vi "Test Normalise.vi"(11 "Test Case In":refnum<class "Vector 2D Tests.lvclass">) -> (0 "error out":errorcluster, 3 "Test Case Out":refnum<class "Vector 2D Tests.lvclass">)   [LabVIEW 2021, in "Vector 2D Tests.lvclass"]
uses:
  Vector 2D Tests.lvclass
  4993e8ee-a06a-463a-9684-69129f64d5ce.vi
  Re-use Libraries/Vector 2D/Vector 2D.lvclass
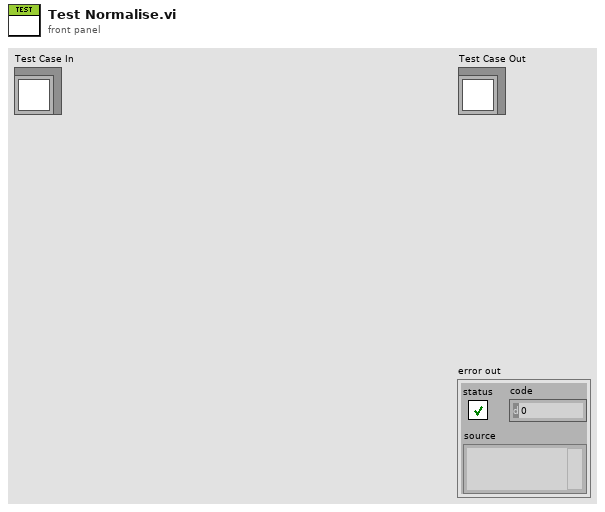
[diagram p1: front panel]
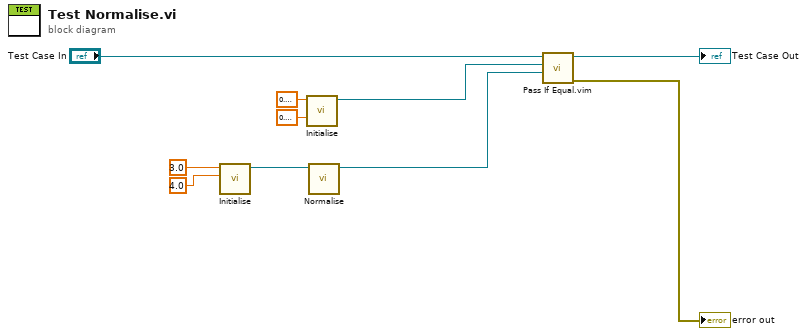
[diagram p0: block diagram]
diagram:
  n1 = call "Initialise.vi"("y"=sgl 4.0, "x"=sgl 3.0) -> ("Vector 2D out"=w9:refnum<class "Vector 2D.lvclass">)  [unwired: 9 in]
  n2 = call "Initialise.vi"("y"=sgl 0.8, "x"=sgl 0.6) -> ("Vector 2D out"=w4:refnum<class "Vector 2D.lvclass">)  [unwired: 9 in]
  n3 = call "Normalise.vi"("Vector 2D in"=w9) -> ("Vector 2D out"=w3:refnum<class "Vector 2D.lvclass">)  [unwired: 10 in]
  n4 = call "Pass If Equal.vim"("Actual"=w3, "Expected"=w4, "LUnit Test Case In"="Test Case In") -> ("error out"=→"error out":errorcluster, "LUnit Test Case Out"=→"Test Case Out":refnum<class "Vector 2D Tests.lvclass">)  [unwired: 7 in]
